vi "WPI_CameraGet Image Data.vi"(8 "error in (no error)":errorcluster, 10 "Image":T1, 11 "CameraDevRef":T2={"Camera Address"="192.168.0.90", "CameraStatus"={"status"=FALSE, "code"=0, "source"=""}}) -> (0 "error out":errorcluster, 1 "Image Data String":string, 2 "Image Out":T1, 3 "CameraDevRef Out":T2)   [LabVIEW 2016]
doc: "Retrieves a specific image from the image data that the camera you specify acquired. Use the Start VI to start acquiring image data from the camera before you use the Get Image VI to retrieve an image. When you run this VI, this VI retrieves the most current snapshot of the image data from the camera.\n\nThis software is licensed. Open the labview\\readme\\WPI Robotics Library Open Source License.txt file for more information."
uses:
  <vilib>/Rock Robotics/WPI/Camera/WPI_CameraDevRef.ctl
  <vilib>/vision/Image Controls.llb/IMAQ Image.ctl
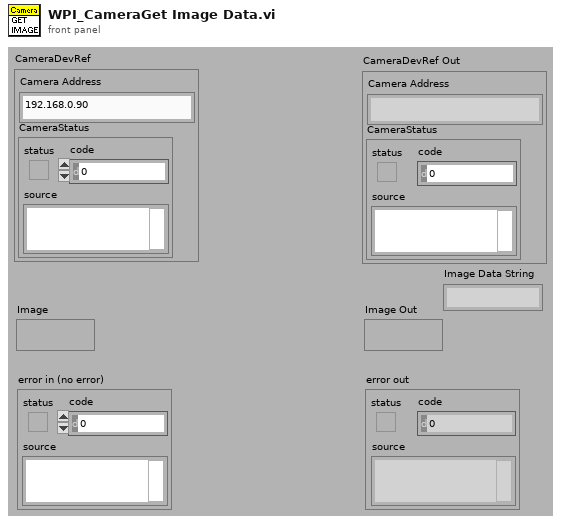
[diagram p1: front panel]
types:
  T1 = typedef "IMAQ Image.ctl" = refnum<image>
  T2 = typedef "WPI_CameraDevRef.ctl" = cluster{"Camera Address":string, "CameraStatus":errorcluster}
  T3 = enum16{"Update Mode", "Get Image", "Get Image Data"}
  T4 = typedef "WPI_CameraFrameRate.ctl" = u32
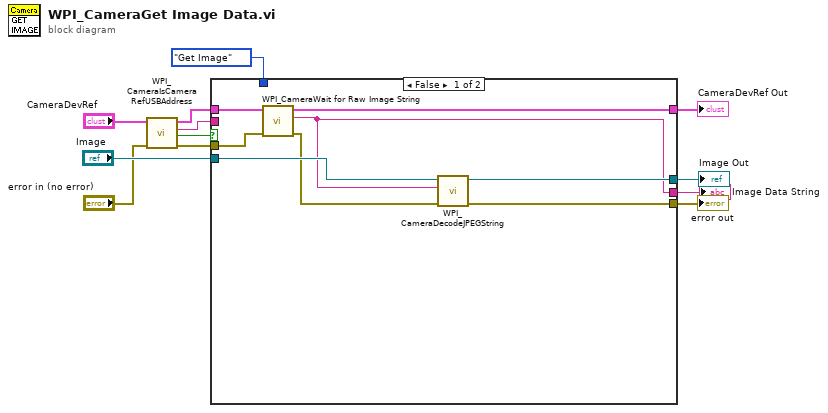
[diagram p0: block diagram]
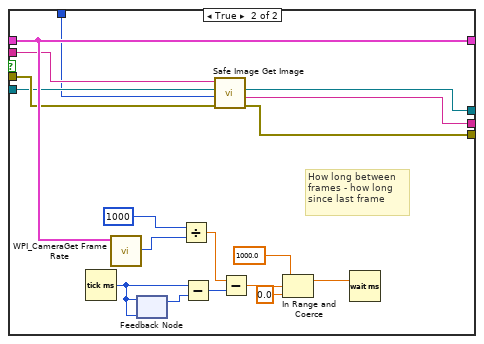
[diagram p2: hidden frame]
diagram:
  n1 = call <vilib>:"WPI_CameraIsCameraRefUSBAddress.vi"("error in (no error)"="error in (no error)", "CameraDevRef"="CameraDevRef") -> ("error out"=w7:errorcluster, "USB?"=w6:bool, "Camera Address Out"=w5:string, "CameraDevRef out"=w3:T2)  [unwired: 6 in]
  n2 = case shown="False" w6 {
    tunnel: "Image" -> [w20 w30]
    tunnel: [w19 w26] -> w11
    tunnel: [w18 w27] -> w10
    tunnel: w3 -> [w16 w34]
    tunnel: [w15 w34] -> w9
    tunnel: w5 -> [_ w29]
    tunnel: w7 -> [w14 w31]
    tunnel: T3."Get Image" ("Operation") -> [_ w28]
    tunnel: [w13 w21] -> w1
    frame False {
      n3 = call <vilib>:"WPI_CameraWait for Raw Image String.vi"("error in (no error)"=w14, "CameraDevRef"=w16) -> ("error out"=w17:errorcluster, "String"=w13:string, "CameraDevRef Out"=w15:T2)  [unwired: 3 in, 4 out]
      n4 = call <vilib>:"WPI_CameraDecodeJPEGString.vi"("error in"=w17, "Compressed Image"=w13, "Image In"=w20) -> ("error out"=w18:errorcluster, "Image Out"=w19:T1)  [unwired: 3 out]
    }
    frame True {
      # "How long between\nframes - how long\nsince last frame"
      n5 = Tick Count (ms)() -> (millisecond timer value=w37:u32)
      n6 = call <vilib>:"WPI_CameraGet Frame Rate.vi"("CameraDevRef"=w34) -> ("Frame Rate (fps)"=w35:T4)  [unwired: 8 in, 2 out]
      n7 = feedback-in #1(w37) -> ()
      n8 = feedback #1(w37) -> (w38:u32)
      n9 = Divide(x=1000, y=w35) -> (x/y=w32:dbl)
      n10 = Subtract(x=w37, y=w38) -> (x-y=w33:u32)
      n11 = call <vilib>:"Safe Image Get Image.vi"("error in"=w31, "Operation"=w28, "Image In"=w30, "Session In"=w29) -> ("error out"=w27:errorcluster, "Image Data String"=w21:string, "Image Out"=w26:T1)  [unwired: 4 in, 1 out]
      n12 = Subtract(x=w32, y=w33) -> (x-y=w25:dbl)
      n13 = In Range and Coerce(upper limit=1000.0, x=w25, lower limit=0.0) -> (coerced(x)=w24:dbl)  [unwired: 1 out]
      n14 = Wait (ms)(milliseconds to wait=w24) -> ()  [unwired: 1 out]
    }
  }
  "CameraDevRef Out" <- w9
  "Image Out" <- w11
  "error out" <- w10
  "Image Data String" <- w1
